vi "calibrateValue.vi"(8 "error in (no error)":errorcluster, 9 "value":string, 10 "channelName":string, 11 "StaticOutputEditor in":refnum<class "StaticOutputEditor.lvclass">) -> (0 "error out":errorcluster, 2 "calibratedValue":dbl, 3 "StaticOutputEditor out":refnum<class "StaticOutputEditor.lvclass">)   [LabVIEW 2011, in "Views.lvlib" / "ScriptEditor.lvlib" / "StaticOutputEditor.lvclass"]
uses:
  StaticOutputEditor.lvclass
  StaticOutputEditor.lvclass/StaticOutputEditor.ctl
  Tools/DatabaseHelpers/Database Objects/ChannelArray/ChannelArray.lvclass
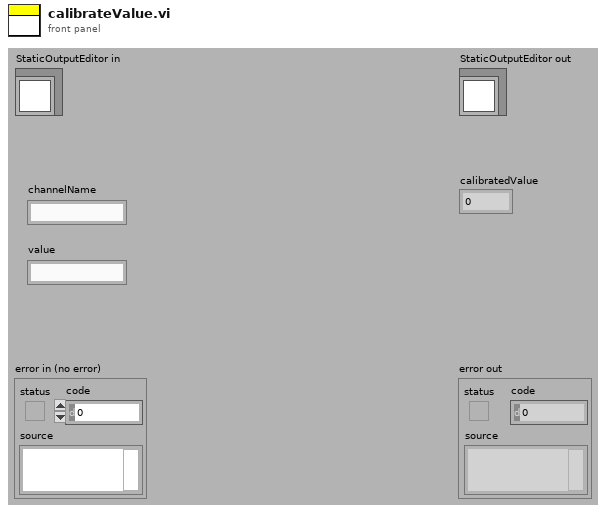
[diagram p1: front panel]
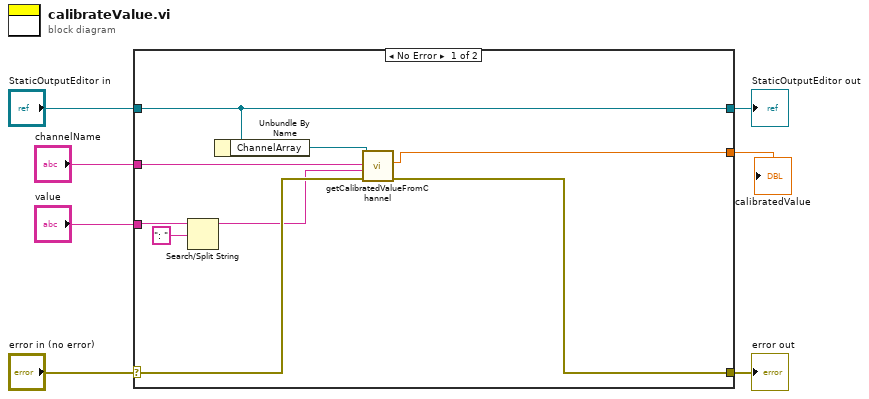
[diagram p0: block diagram]
diagram:
  n1 = case shown="No Error" "error in (no error)" {
    selector: "error in (no error)" -> [w12 w18]
    tunnel: [w11 w18] -> w6
    tunnel: [w16 w17] -> w4
    tunnel: "StaticOutputEditor in" -> [w16 w17]
    tunnel: "channelName" -> [w14 _]
    tunnel: "value" -> [w10 _]
    tunnel: [w13 _] -> w1
    frame No Error {
      n2 = Search/Split String(string=w10, search string/char (-)=": ") -> (substring before match=w9:string)  [unwired: 1 in, 2 out]
      n3 = Unbundle By Name(w16) -> ("ChannelArray"=w15:refnum<class "ChannelArray.lvclass">)
      n4 = call "getCalibratedValueFromChannel.vi"("error in (no error)"=w12, "value"=w9, "channel_name"=w14, "ChannelArray in"=w15) -> ("error out"=w11:errorcluster, "calibratedValue"=w13:dbl)  [unwired: 5 in, 1 out]
    }
    frame Error {
    }
  }
  "error out" <- w6
  "StaticOutputEditor out" <- w4
  "calibratedValue" <- w1
